vi "NI PXI-4110 Programmable Power Supply Ch Page.vi"(8 "error in (no error)":errorcluster, 11 "Node Ptr":T4 format="%.0x") -> (0 "error out":errorcluster)   [LabVIEW 2018, in "NI PXI-4110 Programmable Power Supply Custom Device.lvlib"]
uses:
  NI PXI-4110 Programmable Power Supply Custom Device.lvlib
  <vilib>/NI Veristand/Custom Device API/Custom Device Item Ref.ctl
  IO_Type.ctl
  <instrlib>/niDCPower/nidcpower.llb/niDCPower Sense.ctl
  4110_Channel #.ctl
  4110_Global.vi
  <vilib>/NI Veristand/Custom Device API/Get Item Property (Boolean).vi
  <vilib>/NI Veristand/Custom Device API/Get Item Property (U16).vi
  <vilib>/NI Veristand/Custom Device API/Get Item Property (Double).vi
  <vilib>/NI Veristand/Custom Device API/Get Item Property (I32).vi
  <vilib>/NI Veristand/Custom Device API/Set Item Property (I32).vi
  <vilib>/NI Veristand/Custom Device API/Set Item Property (U16).vi
  <vilib>/NI Veristand/Custom Device API/Set Item Property (Double).vi
  <vilib>/NI VeriStand/Custom Device API/Custom Device API.lvlib
panel:
  in  "Channel #":T1
  in  "Voltage Limit":dbl caption="Range (0-6V)" format="%.4f"
  in  "Initial Current Value":dbl caption="Range (0.01 -1A)" format="%.4f"
  in  "Current Limit":dbl caption="Range (0.01-1A)" format="%.4f"
  in  "sense":T2=1008 caption="Sense" items=["Local"=1008, "Remote"=1009]
  in  "IO Type":T3
  in  "Initial Voltage Value":dbl caption="Range (0-6V)" format="%_4f"
  in  "Name":string
  in  "Header":cluster{"Section Name":string}={"Section Name"="PXI-4110  Settings"}
  in  "Description":string
  in  "Delete":bool
  # "Voltage  IO Settings"
  # "Current IO Settings"
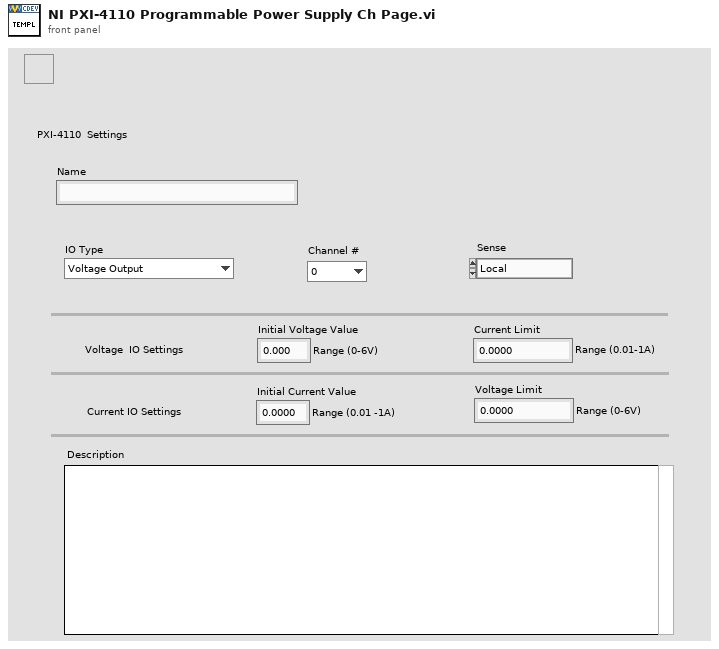
[diagram p1: front panel]
types:
  T1 = typedef "NI PXI-4110 Programmable Power Supply Custom Device.lvlib/4110_Channel #.ctl" = enum16{"0", "1", "2"}
  T2 = typedef "niDCPower Sense.ctl" = i32
  T3 = typedef "NI PXI-4110 Programmable Power Supply Custom Device.lvlib/IO_Type.ctl" = enum16{"Voltage Output", "Current Output"}
  T4 = typedef "Custom Device API.lvlib/Custom Device Item Ref.ctl" = u64
  T5 = enum8{"Enabled", "Disabled", "Disabled and Grayed Out"}
  T6 = cluster{"V_min":dbl, "V_max":dbl, "I_min":dbl, "I_max":dbl}
  T7 = typedef "Custom Device API.lvlib/Custom Device Item Info.ctl" = cluster{"Name":string, "Is Channel":bool, "GUID":string, "Is Waveform":bool}
  T8 = typedef "Custom Device API.lvlib/Custom Device Commands.ctl" = enum16{"Default", "Item renamed", "Shutdown", "Dynamic button pressed"}
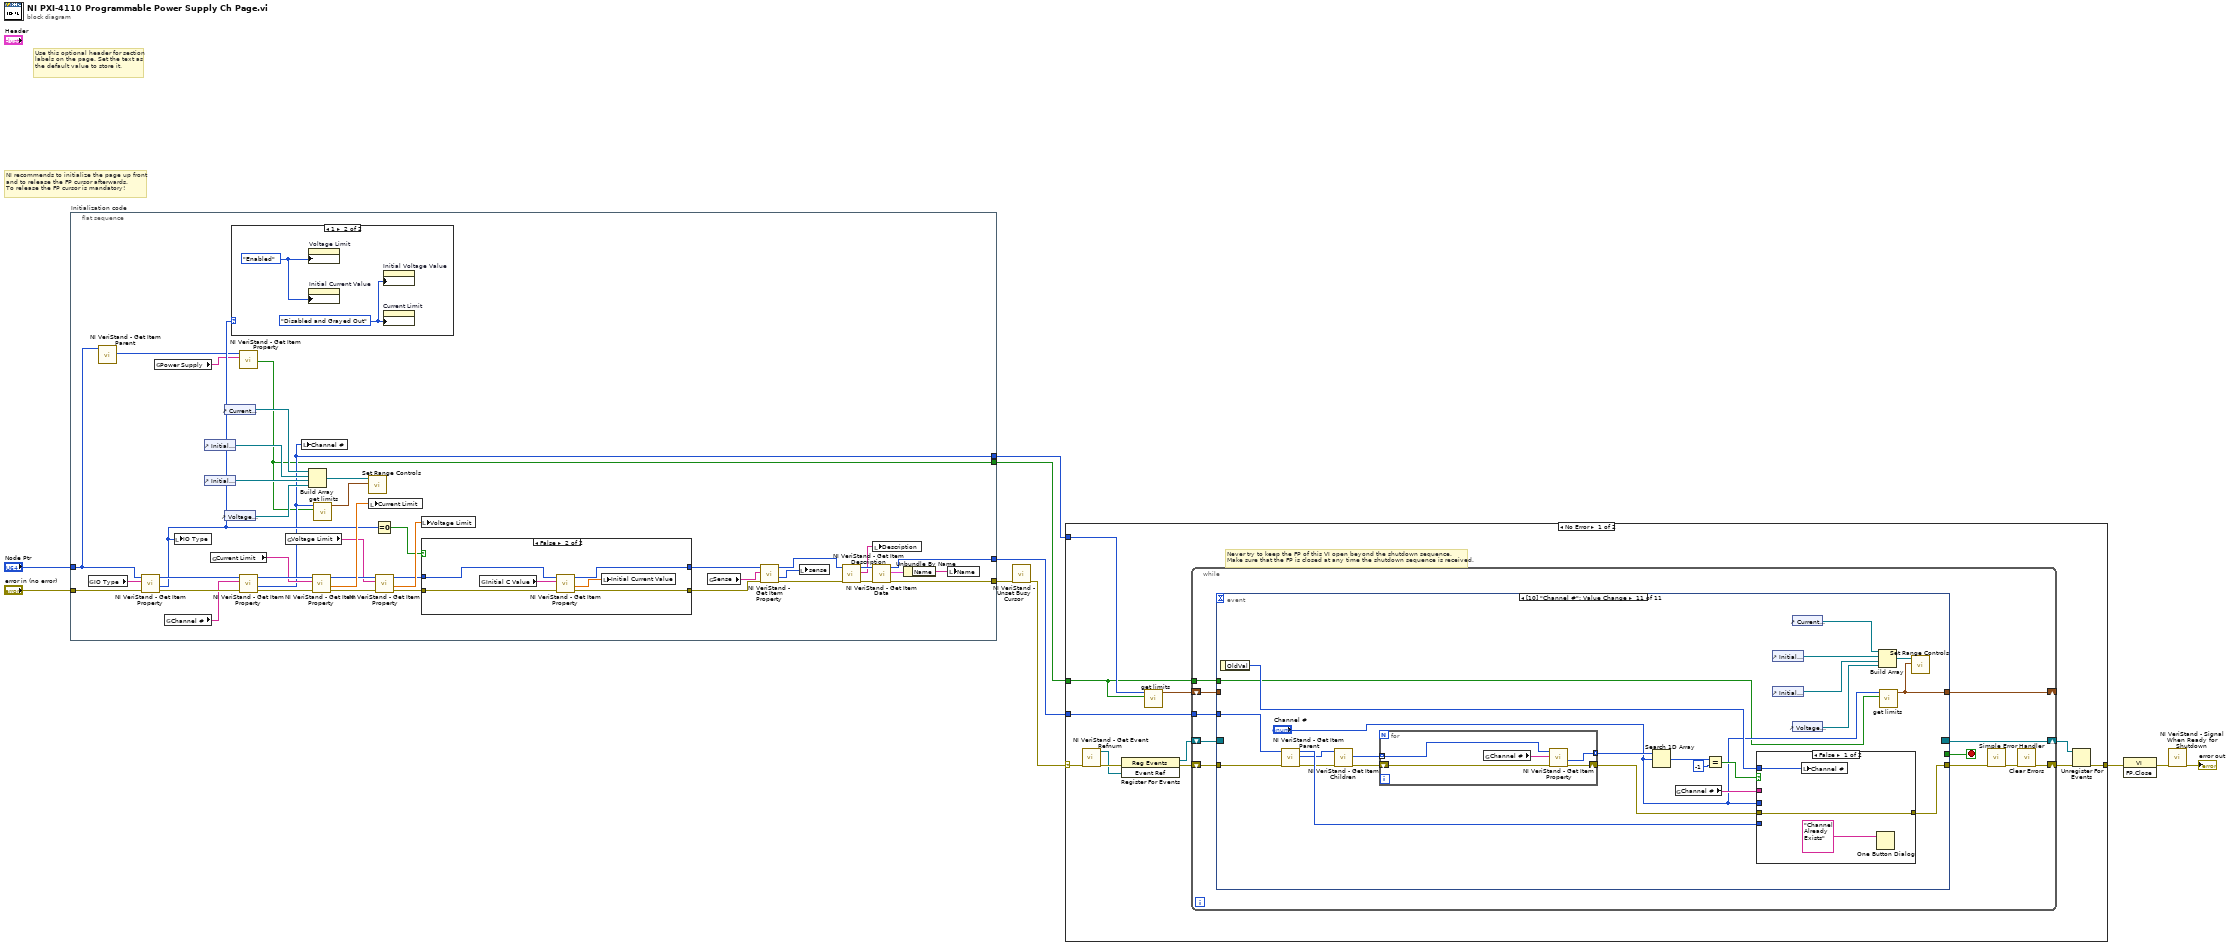
[diagram p0: block diagram]
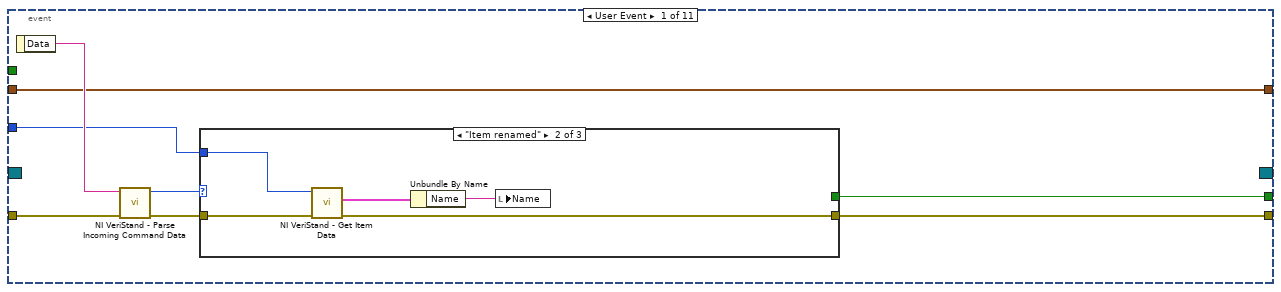
[diagram p2: hidden frame]
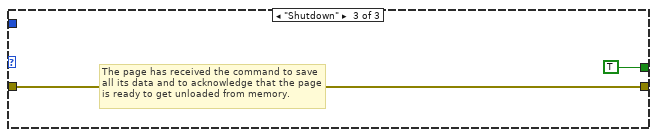
[diagram p4: hidden frame]
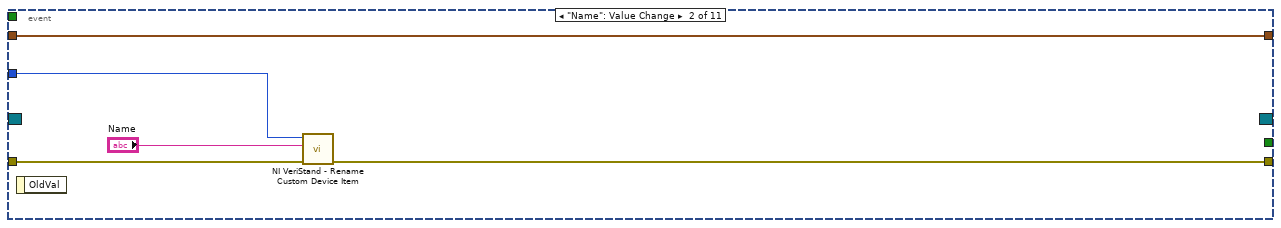
[diagram p5: hidden frame]
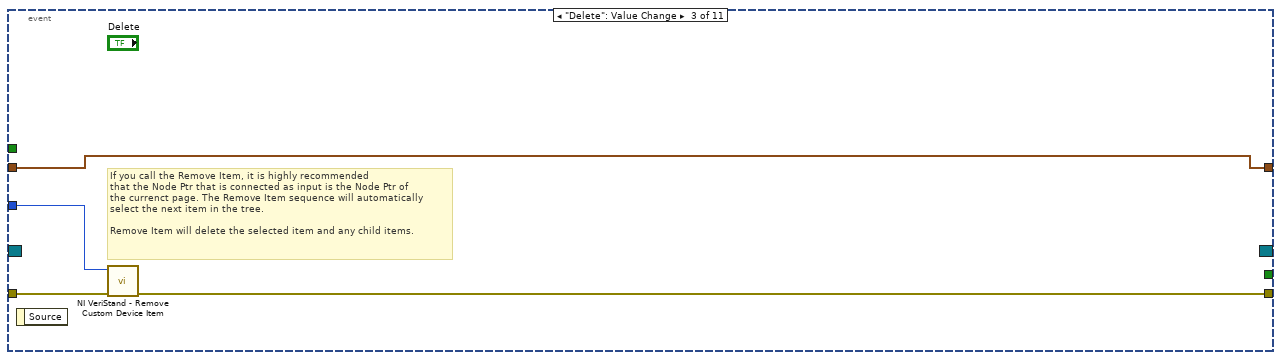
[diagram p6: hidden frame]
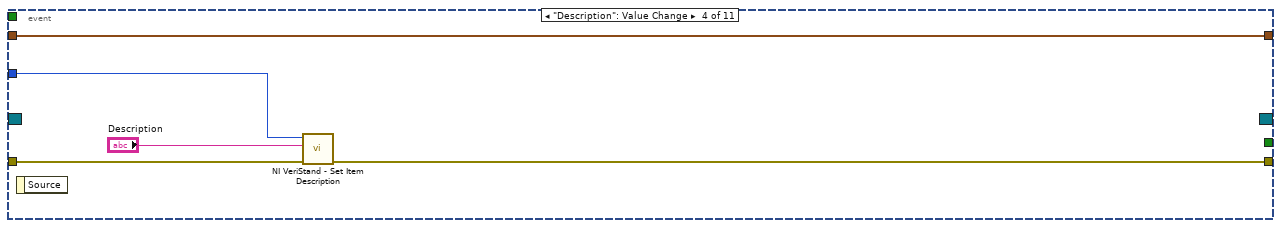
[diagram p7: hidden frame]
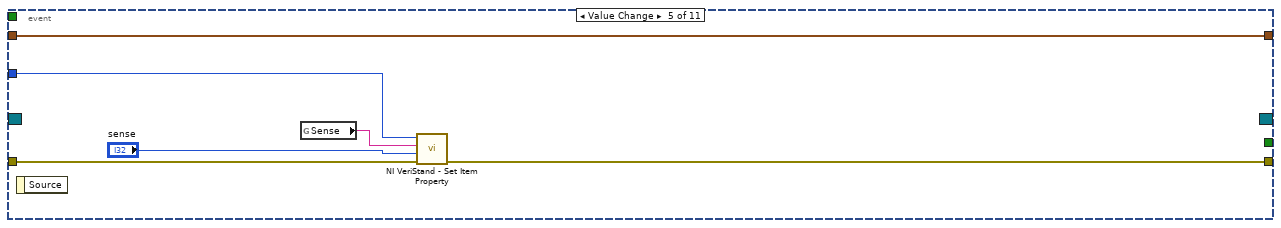
[diagram p8: hidden frame]
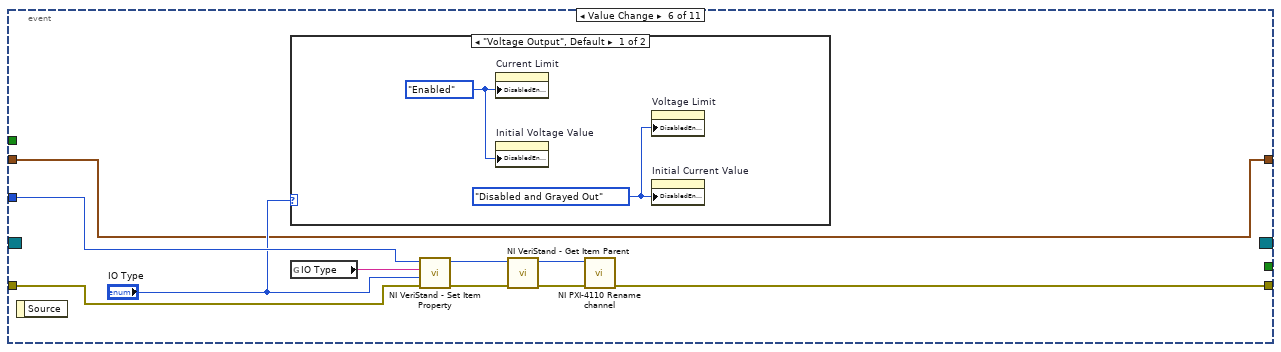
[diagram p9: hidden frame]
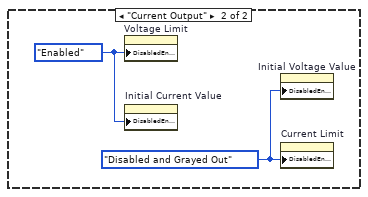
[diagram p10: hidden frame]
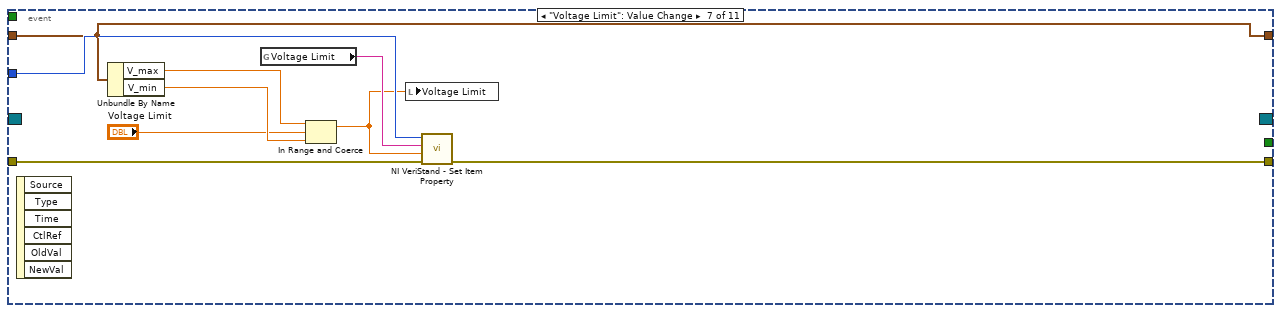
[diagram p11: hidden frame]
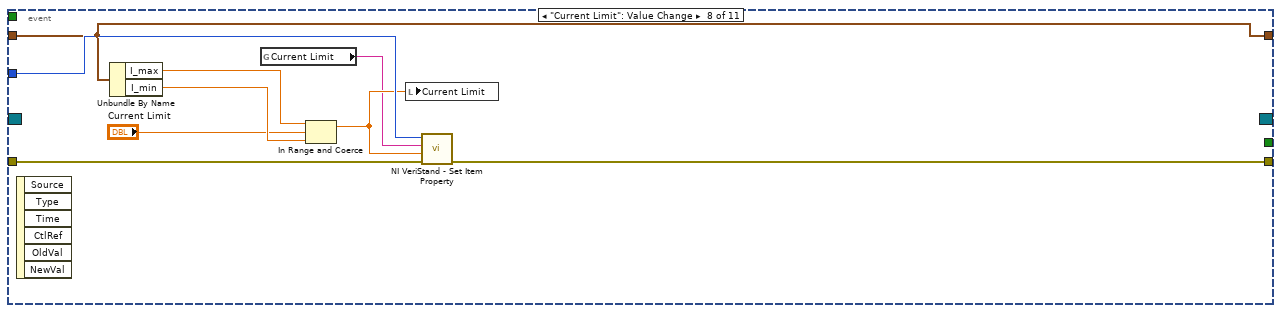
[diagram p12: hidden frame]
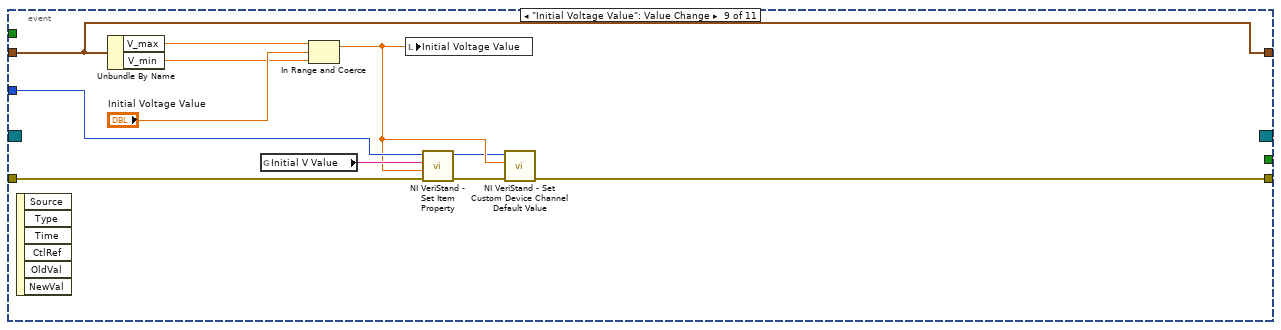
[diagram p13: hidden frame]
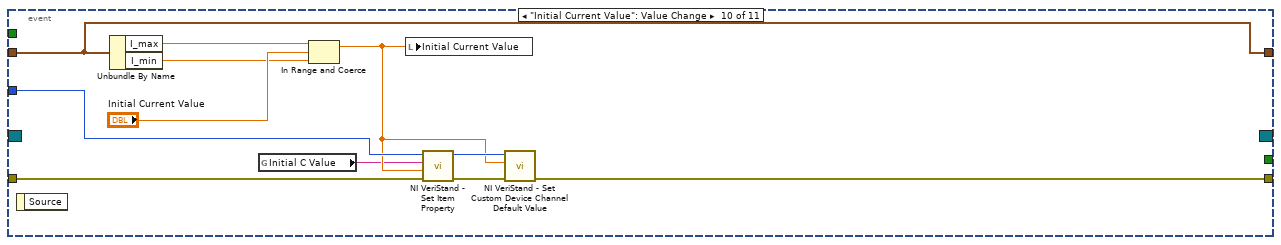
[diagram p14: hidden frame]
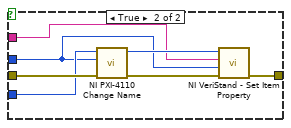
[diagram p15: hidden frame]
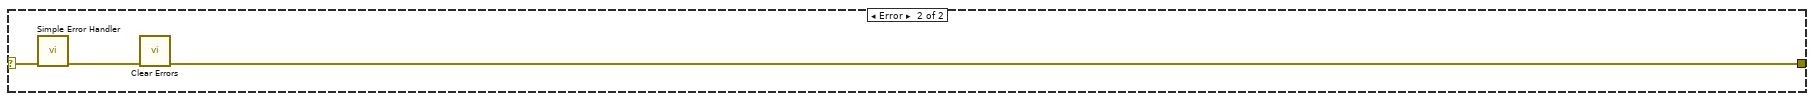
[diagram p16: hidden frame]
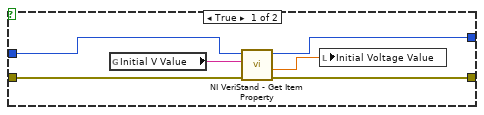
[diagram p17: hidden frame]
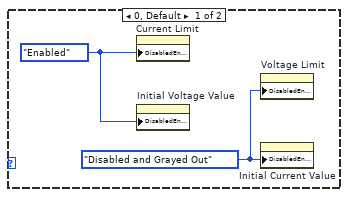
[diagram p18: hidden frame]
diagram:
  # "Use this optional header for section labels on the page. Set the text as the default value to store it."
  # "NI recommends to initialize the page up front\nand to release the FP cursor afterwards.\nTo release the FP cursor is mandatory!"
  n1 = flat-sequence "Initialization code" {
    tunnel: "error in (no error)" -> [w44]
    tunnel: "Node Ptr" -> [w21]
    tunnel: [w46] -> w6
    tunnel: [w51] -> w4
    tunnel: [w12] -> w2
    tunnel: [w11] -> w1
    frame #0 {
      n2 = global read "4110_Global.vi" "IO Type"() -> (w43:string)
      n3 = call <vilib>:"NI VeriStand - Get Item Parent.vi"("Item Ref in"=w21) -> ("Parent Ref"=w19:T4)  [unwired: 7 in, 3 out]
      n4 = call-poly <vilib>:"NI VeriStand - Get Item Property.vi"("error in (no error)"=w44, "Property Name"=w43, "Item Ref in"=w21) -> ("error out"=w42:errorcluster, "Value"=w23:u16, "Item Ref out"=w41:T4)  [unwired: 5 in, 1 out]
      n5 = global read "4110_Global.vi" "Power Supply"() -> (w20:string)
      n6 = global read "4110_Global.vi" "Channel #"() -> (w40:string)
      n7 = local write "IO Type"(w23) -> ()
      n8 = control-ref of="Initial Current Value"() -> (w15:refnum<vi>)
      n9 = control-ref of="Initial Voltage Value"() -> (w16:refnum<vi>)
      n10 = global read "4110_Global.vi" "Current Limit"() -> (w37:string)
      n11 = control-ref of="Current Limit"() -> (w14:refnum<vi>)
      n12 = control-ref of="Voltage Limit"() -> (w17:refnum<vi>)
      n13 = case shown="1" w23 {
        frame 0, Default {
          w64 = T5."Enabled" ("Disabled")
          w65 = T5."Disabled and Grayed Out" ("Disabled")
          n14 = property on="Current Limit" class="DigNum (strict)"("DisabledEnum"=w64) -> ()  [unwired: 2 in, 2 out]
          n15 = property on="Initial Voltage Value" class="DigNum (strict)"("DisabledEnum"=w64) -> ()  [unwired: 2 in, 2 out]
          n16 = property on="Voltage Limit" class="DigNum (strict)"("DisabledEnum"=w65) -> ()  [unwired: 2 in, 2 out]
          n17 = property on="Initial Current Value" class="DigNum (strict)"("DisabledEnum"=w65) -> ()  [unwired: 2 in, 2 out]
        }
        frame 1 {
          w66 = T5."Enabled" ("Disabled")
          w67 = T5."Disabled and Grayed Out" ("Disabled")
          n18 = property on="Voltage Limit" class="DigNum (strict)"("DisabledEnum"=w66) -> ()  [unwired: 2 in, 2 out]
          n19 = property on="Initial Current Value" class="DigNum (strict)"("DisabledEnum"=w66) -> ()  [unwired: 2 in, 2 out]
          n20 = property on="Initial Voltage Value" class="DigNum (strict)"("DisabledEnum"=w67) -> ()  [unwired: 2 in, 2 out]
          n21 = property on="Current Limit" class="DigNum (strict)"("DisabledEnum"=w67) -> ()  [unwired: 2 in, 2 out]
        }
      }
      n22 = call-poly <vilib>:"NI VeriStand - Get Item Property.vi"("Property Name"=w20, "Item Ref in"=w19) -> ("Value"=w11:bool)  [unwired: 6 in, 3 out]
      n23 = call-poly <vilib>:"NI VeriStand - Get Item Property.vi"("error in (no error)"=w42, "Property Name"=w40, "Item Ref in"=w41) -> ("error out"=w38:errorcluster, "Value"=w12:u16, "Item Ref out"=w39:T4)  [unwired: 5 in, 1 out]
      n24 = global read "4110_Global.vi" "Voltage Limit"() -> (w33:string)
      n25 = local write "Channel #"(w12) -> ()
      n26 = Build Array(w14, w15, w16, w17) -> (w18:refnum<vi>[])
      n27 = call-poly <vilib>:"NI VeriStand - Get Item Property.vi"("error in (no error)"=w38, "Property Name"=w37, "Item Ref in"=w39) -> ("error out"=w35:errorcluster, "Value"=w36:dbl, "Item Ref out"=w34:T4)  [unwired: 5 in, 1 out]
      n28 = call "get limits.vi"("External Supply?"=w11, "Channel #"=w12) -> ("output cluster"=w13:T6)  [unwired: 9 in]
      n29 = call "Set Range Controls.vi"("Ranges"=w13, "Reference Array"=w18) -> ()  [unwired: 10 in]
      n30 = local write "Current Limit"(w36) -> ()
      n31 = Equal To 0?(x=w23) -> (x = 0?=w22:bool)
      n32 = call-poly <vilib>:"NI VeriStand - Get Item Property.vi"("error in (no error)"=w35, "Property Name"=w33, "Item Ref in"=w34) -> ("error out"=w30:errorcluster, "Value"=w32:dbl, "Item Ref out"=w31:T4)  [unwired: 5 in, 1 out]
      n33 = local write "Voltage Limit"(w32) -> ()
      n34 = case shown="False" w22 {
        tunnel: w31 -> [w57 w63]
        tunnel: w30 -> [w56 w62]
        tunnel: [w55 w61] -> w28
        tunnel: [w54 w60] -> w27
        frame True {
          n35 = global read "4110_Global.vi" "Initial V Value"() -> (w53:string)
          n36 = call-poly <vilib>:"NI VeriStand - Get Item Property.vi"("error in (no error)"=w56, "Property Name"=w53, "Item Ref in"=w57) -> ("error out"=w55:errorcluster, "Value"=w52:dbl, "Item Ref out"=w54:T4)  [unwired: 5 in, 1 out]
          n37 = local write "Initial Voltage Value"(w52) -> ()
        }
        frame False {
          n38 = global read "4110_Global.vi" "Initial C Value"() -> (w59:string)
          n39 = call-poly <vilib>:"NI VeriStand - Get Item Property.vi"("error in (no error)"=w62, "Property Name"=w59, "Item Ref in"=w63) -> ("error out"=w61:errorcluster, "Value"=w58:dbl, "Item Ref out"=w60:T4)  [unwired: 5 in, 1 out]
          n40 = local write "Initial Current Value"(w58) -> ()
        }
      }
      n41 = global read "4110_Global.vi" "Sense"() -> (w26:string)
      n42 = call-poly <vilib>:"NI VeriStand - Get Item Property.vi"("error in (no error)"=w28, "Property Name"=w26, "Item Ref in"=w27) -> ("error out"=w24:errorcluster, "Value"=w29:i32, "Item Ref out"=w25:T4)  [unwired: 5 in, 1 out]
      n43 = local write "sense"(w29) -> ()
      n44 = call <vilib>:"NI VeriStand - Get Item Description.vi"("error in (no error)"=w24, "Item Ref in"=w25) -> ("error out"=w48:errorcluster, "Description"=w49:string, "Item Ref out"=w50:T4)  [unwired: 7 out]
      n45 = local write "Description"(w49) -> ()
      n46 = call <vilib>:"NI VeriStand - Get Item Data.vi"("error in (no error)"=w48, "Item Ref in"=w50) -> ("error out"=w46:errorcluster, "Item Info"=w47:T7, "Item Ref out"=w51:T4)  [unwired: 7 out]
      n47 = Unbundle By Name(w47) -> ("Name"=w45:string)
      n48 = local write "Name"(w45) -> ()
    }
  }
  n49 = call <vilib>:"NI VeriStand - Unset Busy Cursor.vi"("error in (no error)"=w6) -> ("error out"=w5:errorcluster)  [unwired: 10 out]
  n50 = case shown="No Error" w5 {
    selector: w5 -> [w71 w221]
    tunnel: [w76 w219] -> w10
    tunnel: w4 -> [w72 _]
    tunnel: w2 -> [w70 _]
    tunnel: w1 -> [w68 _]
    frame No Error {
      # "Never try to keep the FP of this VI open beyond the shutdown sequence.\nMake sure that the FP is closed at any time the shutdown sequence is received."
      n51 = call <vilib>:"NI VeriStand - Get Event Refnum.vi"("error in (no error)"=w71) -> ("error out"=w79:errorcluster, "Event Ref"=w75:refnum<user-event>)  [unwired: 9 out]
      n52 = register-events(error in=w79, w75) -> (reference out=w73:refnum<event-registration>, error out=w74:errorcluster)  [unwired: 1 in]
      n53 = call "get limits.vi"("External Supply?"=w68, "Channel #"=w70) -> ("output cluster"=w69:T6)  [unwired: 9 in]
      n54 = while {
        tunnel: w72 -> [w86]
        shift-right: [w83] -> w77
        shift-left: w74 -> [w89]
        shift-right: [w90] -> w78
        shift-left: w73 -> [w88]
        shift-right: [w82] -> _
        shift-left: w69 -> [w81]
        tunnel: w68 -> [w80]
        stop <- w87 stop-if-true
        n55 = event shown="[10] \"Channel #\": Value Change" {
          selector: w88 -> [_ _ _ _ _ _ _ _ _ _ _]
          dyn-events: [_ _ _ _ _ _ _ _ _ _ _] -> w90
          timeout: _ -> [_ _ _ _ _ _ _ _ _ _ _]
          tunnel: w89 -> [w98 w111 w115 w119 w126 w135 w148 w157 w168 w179 w190]
          tunnel: [w94 _ _ _ _ _ _ _ _ _ _] -> w87
          tunnel: [w93 w110 w114 w118 w125 w129 w147 w156 w165 w177 w189] -> w85
          tunnel: w86 -> [w92 w109 w113 w120 w124 w136 w149 w158 w169 w180 w191]
          tunnel: [w91 w107 w112 w116 w121 w127 w145 w153 w161 w174 w181] -> w82
          tunnel: w81 -> [w91 w107 w112 w116 w121 w127 w145 w153 w161 w174 _]
          tunnel: w80 -> [_ _ _ _ _ _ _ _ _ _ w187]
          event User Event {
            n56 = event-data() -> ("Data"=w97:string)  [unwired: 1 out]
            n57 = call <vilib>:"NI VeriStand - Parse Incoming Command Data.vi"("error in (no error)"=w98, "Incoming data"=w97) -> ("error out"=w96:errorcluster, "Action"=w95:T8)  [unwired: 8 out]
            n58 = case shown="\"Item renamed\"" w95 {
              tunnel: w96 -> [w99 w104 w105]
              tunnel: [_ _ TRUE] -> w94
              tunnel: [w99 w101 w105] -> w93
              tunnel: w92 -> [_ w103 _]
              frame "Default", Default {
              }
              frame "Item renamed" {
                n59 = call <vilib>:"NI VeriStand - Get Item Data.vi"("error in (no error)"=w104, "Item Ref in"=w103) -> ("error out"=w101:errorcluster, "Item Info"=w102:T7)  [unwired: 8 out]
                n60 = Unbundle By Name(w102) -> ("Name"=w100:string)
                n61 = local write "Name"(w100) -> ()
              }
              frame "Shutdown" {
                # "The page has received the command to save all its data and to acknowledge that the page is ready to get unloaded from memory."
              }
            }
          }
          event "Name": Value Change {
            n62 = event-data() -> ()  [unwired: 2 out]
            n63 = call <vilib>:"NI VeriStand - Rename Custom Device Item.vi"("error in (no error)"=w111, "New Name"="Name", "Item Ref in"=w109) -> ("error out"=w110:errorcluster)  [unwired: 1 in, 7 out]
          }
          event "Delete": Value Change {
            # "If you call the Remove Item, it is highly recommended\nthat the Node Ptr that is connected as input is the Node Ptr of\nthe currenct page. The Remove Item sequence will automatically\nselect the next item in the tree.\n\nRemove Item will delete the selected item and any child items."
            n64 = event-data() -> ()  [unwired: 2 out]
            n65 = call <vilib>:"NI VeriStand - Remove Custom Device Item.vi"("error in (no error)"=w115, "Item Ref in"=w113) -> ("error out"=w114:errorcluster)  [unwired: 1 in, 8 out]
          }
          event "Description": Value Change {
            n66 = event-data() -> ()  [unwired: 2 out]
            n67 = call <vilib>:"NI VeriStand - Set Item Description.vi"("error in (no error)"=w119, "Description"="Description", "Item Ref in"=w120) -> ("error out"=w118:errorcluster)  [unwired: 8 out]
          }
          event Value Change {
            n68 = event-data() -> ()  [unwired: 2 out]
            n69 = global read "4110_Global.vi" "Sense"() -> (w123:string)
            n70 = call-poly <vilib>:"NI VeriStand - Set Item Property.vi"("error in (no error)"=w126, "Value"="sense", "Property Name"=w123, "Item Ref in"=w124) -> ("error out"=w125:errorcluster)  [unwired: 5 in, 2 out]
          }
          event Value Change {
            n71 = event-data() -> ()  [unwired: 2 out]
            n72 = case shown="\"Voltage Output\", Default" "IO Type" {
              frame "Voltage Output", Default {
                w137 = T5."Enabled" ("Disabled")
                w138 = T5."Disabled and Grayed Out" ("Disabled")
                n73 = property on="Current Limit" class="DigNum (strict)"("DisabledEnum"=w137) -> ()  [unwired: 2 in, 2 out]
                n74 = property on="Initial Voltage Value" class="DigNum (strict)"("DisabledEnum"=w137) -> ()  [unwired: 2 in, 2 out]
                n75 = property on="Voltage Limit" class="DigNum (strict)"("DisabledEnum"=w138) -> ()  [unwired: 2 in, 2 out]
                n76 = property on="Initial Current Value" class="DigNum (strict)"("DisabledEnum"=w138) -> ()  [unwired: 2 in, 2 out]
              }
              frame "Current Output" {
                w139 = T5."Enabled" ("Disabled")
                w140 = T5."Disabled and Grayed Out" ("Disabled")
                n77 = property on="Voltage Limit" class="DigNum (strict)"("DisabledEnum"=w139) -> ()  [unwired: 2 in, 2 out]
                n78 = property on="Initial Current Value" class="DigNum (strict)"("DisabledEnum"=w139) -> ()  [unwired: 2 in, 2 out]
                n79 = property on="Initial Voltage Value" class="DigNum (strict)"("DisabledEnum"=w140) -> ()  [unwired: 2 in, 2 out]
                n80 = property on="Current Limit" class="DigNum (strict)"("DisabledEnum"=w140) -> ()  [unwired: 2 in, 2 out]
              }
            }
            n81 = global read "4110_Global.vi" "IO Type"() -> (w134:string)
            n82 = call-poly <vilib>:"NI VeriStand - Set Item Property.vi"("error in (no error)"=w135, "Value"="IO Type", "Property Name"=w134, "Item Ref in"=w136) -> ("error out"=w132:errorcluster, "Item Ref out"=w130:T4)  [unwired: 5 in, 1 out]
            n83 = call <vilib>:"NI VeriStand - Get Item Parent.vi"("error in (no error)"=w132, "Item Ref in"=w130) -> ("error out"=w128:errorcluster, "Item Ref out"=w131:T4)  [unwired: 6 in, 2 out]
            n84 = call "NI PXI-4110 Rename channel.vi"("error in (no error)"=w128, "Node Ptr"=w131) -> ("error out"=w129:errorcluster)  [unwired: 8 in, 1 out]
          }
          event "Voltage Limit": Value Change {
            n85 = event-data() -> ()  [unwired: 7 out]
            n86 = Unbundle By Name(w145) -> ("V_max"=w144:dbl, "V_min"=w143:dbl)
            n87 = global read "4110_Global.vi" "Voltage Limit"() -> (w146:string)
            n88 = In Range and Coerce(upper limit=w144, x="Voltage Limit", lower limit=w143) -> (coerced(x)=w141:dbl)  [unwired: 1 out]
            n89 = local write "Voltage Limit"(w141) -> ()
            n90 = call-poly <vilib>:"NI VeriStand - Set Item Property.vi"("error in (no error)"=w148, "Value"=w141, "Property Name"=w146, "Item Ref in"=w149) -> ("error out"=w147:errorcluster)  [unwired: 5 in, 2 out]
          }
          event "Current Limit": Value Change {
            n91 = event-data() -> ()  [unwired: 7 out]
            n92 = Unbundle By Name(w153) -> ("I_max"=w155:dbl, "I_min"=w154:dbl)
            n93 = global read "4110_Global.vi" "Current Limit"() -> (w150:string)
            n94 = In Range and Coerce(upper limit=w155, x="Current Limit", lower limit=w154) -> (coerced(x)=w151:dbl)  [unwired: 1 out]
            n95 = local write "Current Limit"(w151) -> ()
            n96 = call-poly <vilib>:"NI VeriStand - Set Item Property.vi"("error in (no error)"=w157, "Value"=w151, "Property Name"=w150, "Item Ref in"=w158) -> ("error out"=w156:errorcluster)  [unwired: 5 in, 2 out]
          }
          event "Initial Voltage Value": Value Change {
            n97 = event-data() -> ()  [unwired: 7 out]
            n98 = Unbundle By Name(w161) -> ("V_max"=w160:dbl, "V_min"=w159:dbl)
            n99 = global read "4110_Global.vi" "Initial V Value"() -> (w167:string)
            n100 = In Range and Coerce(upper limit=w160, x="Initial Voltage Value", lower limit=w159) -> (coerced(x)=w164:dbl)  [unwired: 1 out]
            n101 = local write "Initial Voltage Value"(w164) -> ()
            n102 = call-poly <vilib>:"NI VeriStand - Set Item Property.vi"("error in (no error)"=w168, "Value"=w164, "Property Name"=w167, "Item Ref in"=w169) -> ("error out"=w166:errorcluster, "Item Ref out"=w163:T4)  [unwired: 5 in, 1 out]
            n103 = call <vilib>:"NI VeriStand - Set Custom Device Channel Default Value.vi"("error in (no error)"=w166, "Default Value"=w164, "Channel Ref in"=w163) -> ("error out"=w165:errorcluster)  [unwired: 7 in, 1 out]
          }
          event "Initial Current Value": Value Change {
            n104 = event-data() -> ()  [unwired: 2 out]
            n105 = Unbundle By Name(w174) -> ("I_max"=w173:dbl, "I_min"=w172:dbl)
            n106 = global read "4110_Global.vi" "Initial C Value"() -> (w170:string)
            n107 = In Range and Coerce(upper limit=w173, x="Initial Current Value", lower limit=w172) -> (coerced(x)=w171:dbl)  [unwired: 1 out]
            n108 = local write "Initial Current Value"(w171) -> ()
            n109 = call-poly <vilib>:"NI VeriStand - Set Item Property.vi"("error in (no error)"=w179, "Value"=w171, "Property Name"=w170, "Item Ref in"=w180) -> ("error out"=w178:errorcluster, "Item Ref out"=w176:T4)  [unwired: 5 in, 1 out]
            n110 = call <vilib>:"NI VeriStand - Set Custom Device Channel Default Value.vi"("error in (no error)"=w178, "Default Value"=w171, "Channel Ref in"=w176) -> ("error out"=w177:errorcluster)  [unwired: 7 in, 1 out]
          }
          event Value Change {
            n111 = event-data() -> ("OldVal"=w193:T1)  [unwired: 1 out]
            n112 = call <vilib>:"NI VeriStand - Get Item Parent.vi"("error in (no error)"=w190, "Item Ref in"=w191) -> ("error out"=w194:errorcluster, "Parent Ref"=w195:T4, "Item Ref out"=w203:T4)  [unwired: 6 in, 1 out]
            n113 = call <vilib>:"NI VeriStand - Get Item Children.vi"("error in (no error)"=w194, "Item Ref in"=w195) -> ("error out"=w197:errorcluster, "Child Refs"=w196:T4[])  [unwired: 6 in, 2 out]
            n114 = for {
              tunnel: w196 -> [w216] mode=indexing
              shift-right: [w217] -> w202
              shift-left: w197 -> [w218]
              tunnel: [w215] -> w198 mode=indexing
              n115 = global read "4110_Global.vi" "Channel #"() -> (w214:string)
              n116 = call-poly <vilib>:"NI VeriStand - Get Item Property.vi"("error in (no error)"=w218, "Property Name"=w214, "Item Ref in"=w216) -> ("error out"=w217:errorcluster, "Value"=w215:u16)  [unwired: 5 in, 2 out]
            }
            n117 = Search 1D Array(1D array=w198, element="Channel #") -> (index of element=w199:i32)  [unwired: 1 in]
            n118 = global read "4110_Global.vi" "Channel #"() -> (w192:string)
            n119 = Equal?(x=w199, y=-1) -> (x = y?=w201:bool)
            n120 = case shown="False" w201 {
              tunnel: w202 -> [w205 w213]
              tunnel: w203 -> [_ w212]
              tunnel: w192 -> [_ w208]
              tunnel: "Channel #" -> [_ w207]
              tunnel: [w205 w210] -> w189
              tunnel: w193 -> [w206 _]
              frame False {
                n121 = local write "Channel #"(w206) -> ()
                n122 = One Button Dialog(message="Channel Already Exists") -> ()  [unwired: 1 in, 1 out]
              }
              frame True {
                n123 = call "NI PXI-4110 Change Name.vi"("error in (no error)"=w213, "New #"=w207, "Node Ptr"=w212) -> ("error out"=w211:errorcluster, "Node Ptr out"=w209:T4)  [unwired: 7 in]
                n124 = call-poly <vilib>:"NI VeriStand - Set Item Property.vi"("error in (no error)"=w211, "Value"=w207, "Property Name"=w208, "Item Ref in"=w209) -> ("error out"=w210:errorcluster)  [unwired: 5 in, 2 out]
              }
            }
            n125 = control-ref of="Initial Current Value"() -> (w185:refnum<vi>)
            n126 = control-ref of="Initial Voltage Value"() -> (w184:refnum<vi>)
            n127 = control-ref of="Current Limit"() -> (w186:refnum<vi>)
            n128 = control-ref of="Voltage Limit"() -> (w183:refnum<vi>)
            n129 = Build Array(w186, w185, w184, w183) -> (w182:refnum<vi>[])
            n130 = call "get limits.vi"("External Supply?"=w187, "Channel #"="Channel #") -> ("output cluster"=w181:T6)  [unwired: 9 in]
            n131 = call "Set Range Controls.vi"("Ranges"=w181, "Reference Array"=w182) -> ()  [unwired: 10 in]
          }
        }
        n132 = call <vilib>:"Simple Error Handler.vi"("error in (no error)"=w85) -> ("error out"=w84:errorcluster)  [unwired: 1 in, 7 out]
        n133 = call <vilib>:"Clear Errors.vi"("error in (no error)"=w84) -> ("error out"=w83:errorcluster)  [unwired: 1 in, 5 out]
      }
      n134 = Unregister For Events(event registration refnum=w78, error in=w77) -> (error out=w76:errorcluster)
    }
    frame Error {
      n135 = call <vilib>:"Simple Error Handler.vi"("error in (no error)"=w221) -> ("error out"=w220:errorcluster)  [unwired: 1 in, 7 out]
      n136 = call <vilib>:"Clear Errors.vi"("error in (no error)"=w220) -> ("error out"=w219:errorcluster)  [unwired: 1 in, 5 out]
    }
  }
  n137 = invoke class="VI" method="FP.Close"(error in=w10) -> (error out=w9:errorcluster)  [unwired: 2 in, 2 out]
  n138 = call <vilib>:"NI VeriStand - Signal When Ready for Shutdown.vi"("error in (no error)"=w9) -> ("error out"=→"error out":errorcluster)  [unwired: 10 out]
